vi "Dashboard Main.vi"() -> ()   [LabVIEW 2020]
uses:
  <vilib>/event_ctls.llb/eventvkey.ctl
  <vilib>/Rock Robotics/Network Tables/NT Read Numeric Array.vi
  <vilib>/Rock Robotics/WPI/Dashboard/WPI_DashboardLogging Global.vi
panel:
  in  "Camera Settings Right":T1={"Frame Rate"=30, "Compression"=30, "Size"=1, "DB Camera Config"=FALSE} {"Frame Rate" scale=1.0..30.0; "Compression" scale=100.0..-1.0; "Size" items=["640x480", "320x240", "160x120"]}
  in  "Camera Name Right":string(combo)="No Camera Selection"
  out "Camera Perf":string
  in  "Camera Settings":T1={"Frame Rate"=30, "Compression"=30, "Size"=1, "DB Camera Config"=FALSE} {"Frame Rate" scale=1.0..30.0; "Compression" scale=100.0..-1.0; "Size" items=["640x480", "320x240", "160x120"]}
  in  "TCP":refnum<k5>
  in  "Rec Mode":enum32{"Stop", "Record", "Playback"}(radio)
  out "Robot IP":string
  out "Image Message":string="Timeout in Camera Communications"
  in  "Dashboard Tab":T2(tab)
  in  "Select Auto":string(combo)="Select Autonomous ..."
  out "NT Connection":bool
  out "MotorChart R":cluster{"Numeric":dbl, "Numeric":dbl}(graph)
  out "MotorChart L":cluster{"Numeric":dbl, "Numeric":dbl}(graph)
  out "MotorSliders R":cluster{"MotorSlide1":dbl, "MotorSlide2":dbl} {"MotorSlide2" scale=-1.0..1.0 scale format="%#_2e"; "MotorSlide1" scale=-1.0..1.0 scale format="%#_2e"}
  out "MotorSliders L":cluster{"MotorSlide1":dbl, "MotorSlide2":dbl} {"MotorSlide2" scale=-1.0..1.0 scale format="%#_2e"; "MotorSlide1" scale=-1.0..1.0 scale format="%#_2e"}
  out "Gyro":dbl(knob) scale=0.0..360.0
  out "JS1 Z":dbl(slide) scale=-1.0..1.0 scale format="%#_2e"
  out "JS1 Graph":cluster{"X":dbl, "Y":dbl}[](graph)
  out "JS1 Buttons":T3
  out "JS2 Z":dbl(slide) scale=-1.0..1.0 scale format="%#_2e"
  out "JS2 Graph":cluster{"X":dbl, "Y":dbl}[](graph)
  out "JS2 Buttons":T3
  out "Mode":T4(ring)=enum."Auto Disabled"
  out "Right Camera Perf":cluster{"Bandwidth (Mbps)":dbl, "FPS":dbl}
  out "Camera Image Right":T5(plugin-control)
  in  "DB/String 9":string
  in  "DB/String 8":string
  in  "DB/String 7":string
  in  "DB/String 6":string
  in  "DB/String 5":string
  in  "DB/String 4":string
  in  "DB/String 3":string
  in  "DB/String 2":string
  in  "DB/String 1":string
  in  "DB/String 0":string
  in  "DB/Slider 0":dbl(slide) scale=0.0..5.0
  in  "DB/Slider 1":dbl(slide) scale=0.0..5.0
  in  "DB/Slider 2":dbl(slide) scale=0.0..5.0
  in  "DB/Slider 3":dbl(slide) scale=0.0..5.0
  out "DB/LED 3":bool
  out "DB/LED 2":bool
  out "DB/LED 1":bool
  out "DB/LED 0":bool
  in  "DB/Button 3":bool
  in  "DB/Button 2":bool
  in  "DB/Button 1":bool
  in  "DB/Button 0":bool caption="New Name"
  in  "Test Slider":dbl(slide) scale=0.0..100.0 scale format="%#_3g"
  in  "On/Off":bool caption="Solenoid"
  in  "Test Name":u16(ring) items=["Select the test to run..."]
  in  "Test Tree":string(tree)
  in  "Motor":cluster{"Value":dbl, "Enable":bool} {"Value" scale=-1.0..1.0 scale format="%#_3g"}
  out "Progress":T6 {"Test Progress" scale=0.0..100.0}
  in  "Rev/Fwd":cluster{"Forward":bool, "Reverse":bool}
  in  "Test Ring":u16(ring) items=["Monochrome", "Color"]
  in  "CheckList":i32(listbox)
  out "Tree":string(tree)
  out "XY Graph":cluster{"X":dbl, "Y":dbl}[](graph)
  out "Auto Step":T7 {"Arm"."Position" items=["PICKUP", "A", "B", "C"]; "Arm"."Direction" items=["NOTHING", "IN", "OUT"]}
  in  "Auto Steps":i32[](listbox)
  out "Auto Name":string
  out "Confirm Auto Selection":string
  out "Current Step":string
  in  "Auto Definitions":enum32{"Red 1", "Red 2"}(tab)
  in  "Red 1":T8(array[cluster]) {"Arm"."Position" items=["PICKUP", "A", "B", "C"]; "Arm"."Direction" items=["NOTHING", "IN", "OUT"]}
  in  "Red 2":T8(array[cluster]) {"Arm"."Position" items=["PICKUP", "A", "B", "C"]; "Arm"."Direction" items=["NOTHING", "IN", "OUT"]}
  in  "path to PNG file":path
  out "Formatted Strings":cluster{"Name":string, "Value":string}[](array[cluster])
  out "Camera Image":T5(plugin-control)
  out "Background":bool
  in  "Camera Name":string(combo)="No Camera Selection"
  # "HW"
  # "HW"
  # "Joysticks"
  # "Drive Motors"
  # "Front"
  # "Right"
  # "Left"
  # "Back"
  # "This tab is a great place for autonomous settings and robot-specific values.\nPlace controls and indicators inside this tab and match name to\nDashboard Variables on robot. You can also delete this comment."
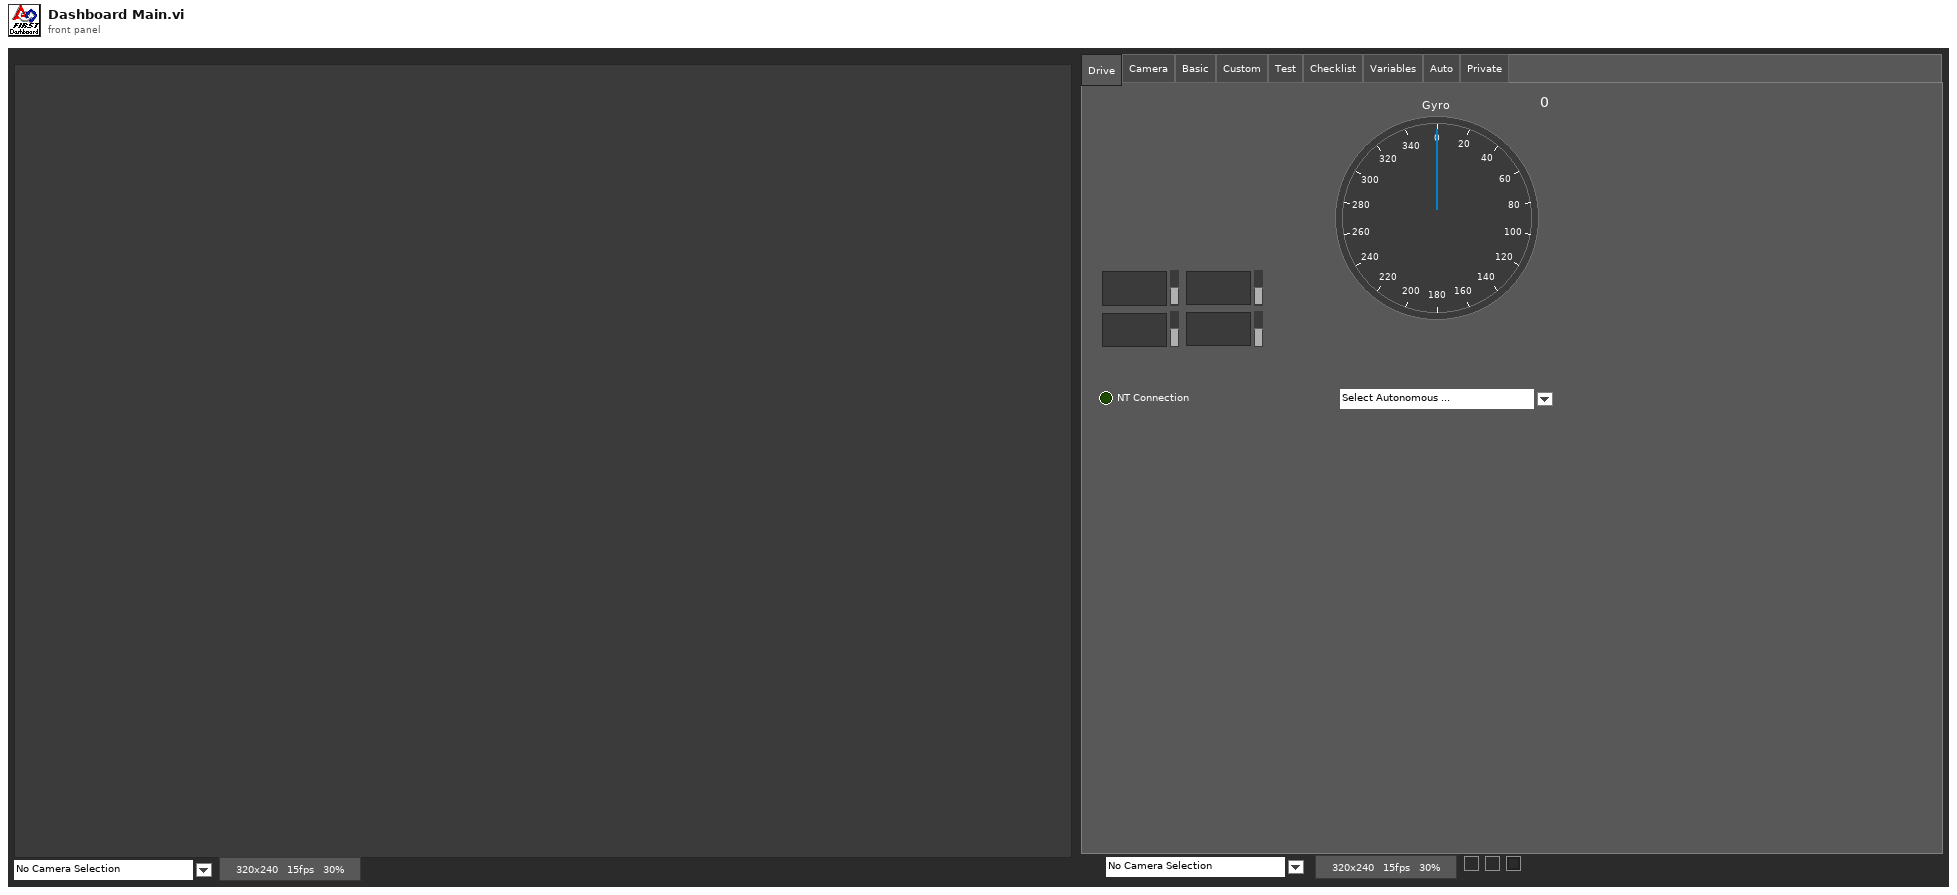
[diagram p1: front panel]
types:
  T1 = cluster{"Frame Rate":i32, "Compression":i32, "Size":u16, "DB Camera Config":bool}
  T2 = enum32{"Drive", "Camera", "Basic", "Custom", "Test", "Checklist", "Variables", "Auto", "Private"}
  T3 = cluster{bool, bool, bool, bool, bool, bool, bool, bool, bool, bool, bool, bool}
  T4 = enum8{"Tele-Op Disabled", "Tele-Op Enabled", "Auto Disabled", "Auto Enabled", "Test Disabled", "Test Enabled", "Disconnected", "No Code", "E-Stop"}
  T5 = typedef "IMAQ Image.ctl" = refnum<image>
  T6 = cluster{"Test Progress":u8, "Test Progress Text":string}
  T7 = cluster{"Step Name":string, "Position Change":cluster{"X":dbl, "Y":dbl, "Rotation":dbl, "Speed":dbl}, "Arm":cluster{"Direction":u16, "Position":u16}}
  T8 = cluster{"Step Name":string, "Position Change":cluster{"X":dbl, "Y":dbl, "Rotation":dbl, "Speed":dbl}, "Arm":cluster{"Direction":u16, "Position":u16}}[]
  T9 = enum32{"Drive", "Camera", "Basic", "Custom", "Test", "Checklist", "Variables"}
  T10 = cluster{"Save Path":path, "Interval (s)":dbl, "Keep":i32}
  T11 = enum32{"Drive", "Camera", "Basic", "Custom", "Test", "Commands", "Checklist", "Variables"}
  T12 = typedef "Image Type" = u32
  T13 = cluster{"Error Strings":string, "Disable Counts":cluster{u16, u16}, "Rail Faults":cluster{u16, u16, u16}, "Robot IP":string, "DB Mode":u8, "Event Info":cluster{"Name":string, "Type":u8, "Number":u16, "Replay":u8}}
  T14 = cluster{"Storage":cluster{"Disk Free":u64, "RAM Block":u32, "RAM free":u32}, "CPU Utilization":cluster{"CPU % ISR":sgl, "CPU % Time Crit":sgl, "CPU % Timed Str":sgl, "CPU % High":sgl, "CPU % Above":sgl, "CPU % Normal":sgl, "CPU % Low":sgl}, "CAN":cluster{"% Bus Utilization":sgl, "Bus Off Cnt":u32, "TX_FIFO Full Cnt":u32, "Receive Error Cnt":u8, "Transmit Error Cnt":u8}, "HID":cluster{"HID Outputs":u32, "Rumble Low":u16, "Rumble High":u16}[]}
  T15 = cluster{"Status bits":cluster{"Test Mode":bool, "Autonomous":bool, "Enabled":bool, "Code Start":bool, "Brownout":bool, "Reserved 2":bool, "Reserved 3":bool, "E-Stop":bool}, "Code Trace":cluster{"Disabled":bool, "TeleOp":bool, "Auto":bool, "Test":bool}, "Controller Type":enum16{"unknown", "cRIO", "roboRio"}, "Code?":enum16{"unknown", "noCode", "code"}, "Battery V":dbl}
  T16 = cluster{"Control Bits":cluster{"TestMode":bool, "Autonomous":bool, "Enabled":bool, "FMS Present":bool, bool, bool, bool, "E-Stop":bool}, "Team Station ":u8, "Countdown":sgl, "Joystick Values":cluster{"Axes":dbl[], "Buttons":bool[], "POVs":i16[]}[]}
  T17 = cluster{"Axes":dbl[], "Buttons":bool[], "POVs":i16[]}[]
  T18 = cluster{"Axes":dbl[], "Buttons":bool[], "POVs":i16[]}
  T19 = cluster{"Buttons[0]":bool, "Buttons[1]":bool, "Buttons[2]":bool, "Buttons[3]":bool, "Buttons[4]":bool, "Buttons[5]":bool, "Buttons[6]":bool, "Buttons[7]":bool, "Buttons[8]":bool, "Buttons[9]":bool, "Buttons[10]":bool, "Buttons[11]":bool}
  T20 = cluster{"Camera Image":refnum<vi>, "Dashboard Tab":refnum<vi>, "Background":refnum<vi>, "Rec Mode":refnum<vi>, "Test Slider":refnum<vi>, "On/Off ":refnum<vi>, "Test Ring":refnum<vi>, "Rev/Fwd":refnum<vi>, "Test Name":refnum<vi>, "Motor":refnum<vi>, "Progress":refnum<vi>, "CheckList":refnum<vi>, "Tree":refnum<vi>, "Test Tree":refnum<vi>, "Camera Settings":refnum<vi>, "Camera Name":refnum<vi>, "Camera Perf":refnum<vi>, "Camera Settings Right":refnum<vi>, "Camera Name Right":refnum<vi>, "Camera Image Right":refnum<vi>}
  T21 = cluster{"Global Rectangle":i32[], "Contours":cluster{"Contour Type":u32, "ROI Type":u32, "Points":i32[]}[]}
  T22 = cluster{"Camera Name":string, string, "Saved DB Images Info":cluster{"Save Path":path, "Interval (s)":dbl, "Keep":i32}}
  T23 = cluster{"Camera Name Right":string, string, "Saved DB Images Info":cluster{"Save Path":path, "Interval (s)":dbl, "Keep":i32}}
  T24 = cluster{"X":dbl, "Y":dbl, "Rotation":dbl, "Speed":dbl}
  T25 = cluster{"Operation":enum16{"Update", "Clear"}, "Color Box":u32}[]
  T26 = typedef "eventvkey.ctl" = enum16{"ASCII", "Enter", "Return", "Shift", "Ctrl", "Alt", "Cmd", "Opt", "Caps", "NumLock", "Clear", "Break", "Up", "Down", "Left", "Right", "Insert", "Delete", "Home", "End", "PageUp", "PageDown", "Escape", "Help", "Pause", "ScrollLock", "F1", "F2", "F3", "F4", "F5", "F6", "F7", "F8", "F9", "F10", "F11", "F12", "F13", "F14", "F15", "F16", "F17", "F18", "F19", "F20", "F21", "F22", "F23", "F24", "Play", "VolumeUp", "VolumeDown", "Mute", "Two Byte Char"}
  T27 = cluster{"Image Size":bool, "Image Type":bool, "Pixel Value":bool, "ROI Information":bool, "Zoom Factor":bool}
  T28 = cluster{"Operation":enum16{"Update", "Clear"}, "Color Box":u32}
  T29 = cluster{"Shift":bool, "Ctrl":bool, "Alt":bool, "Cmd":bool, "Opt":bool}
  T30 = typedef "imagedata.ctl" = cluster{"image type":i32, "image depth":i32, "image":u8[], "mask":u8[], "colors":u32[], "Rectangle":cluster{"left":i16, "top":i16, "right":i16, "bottom":i16}}
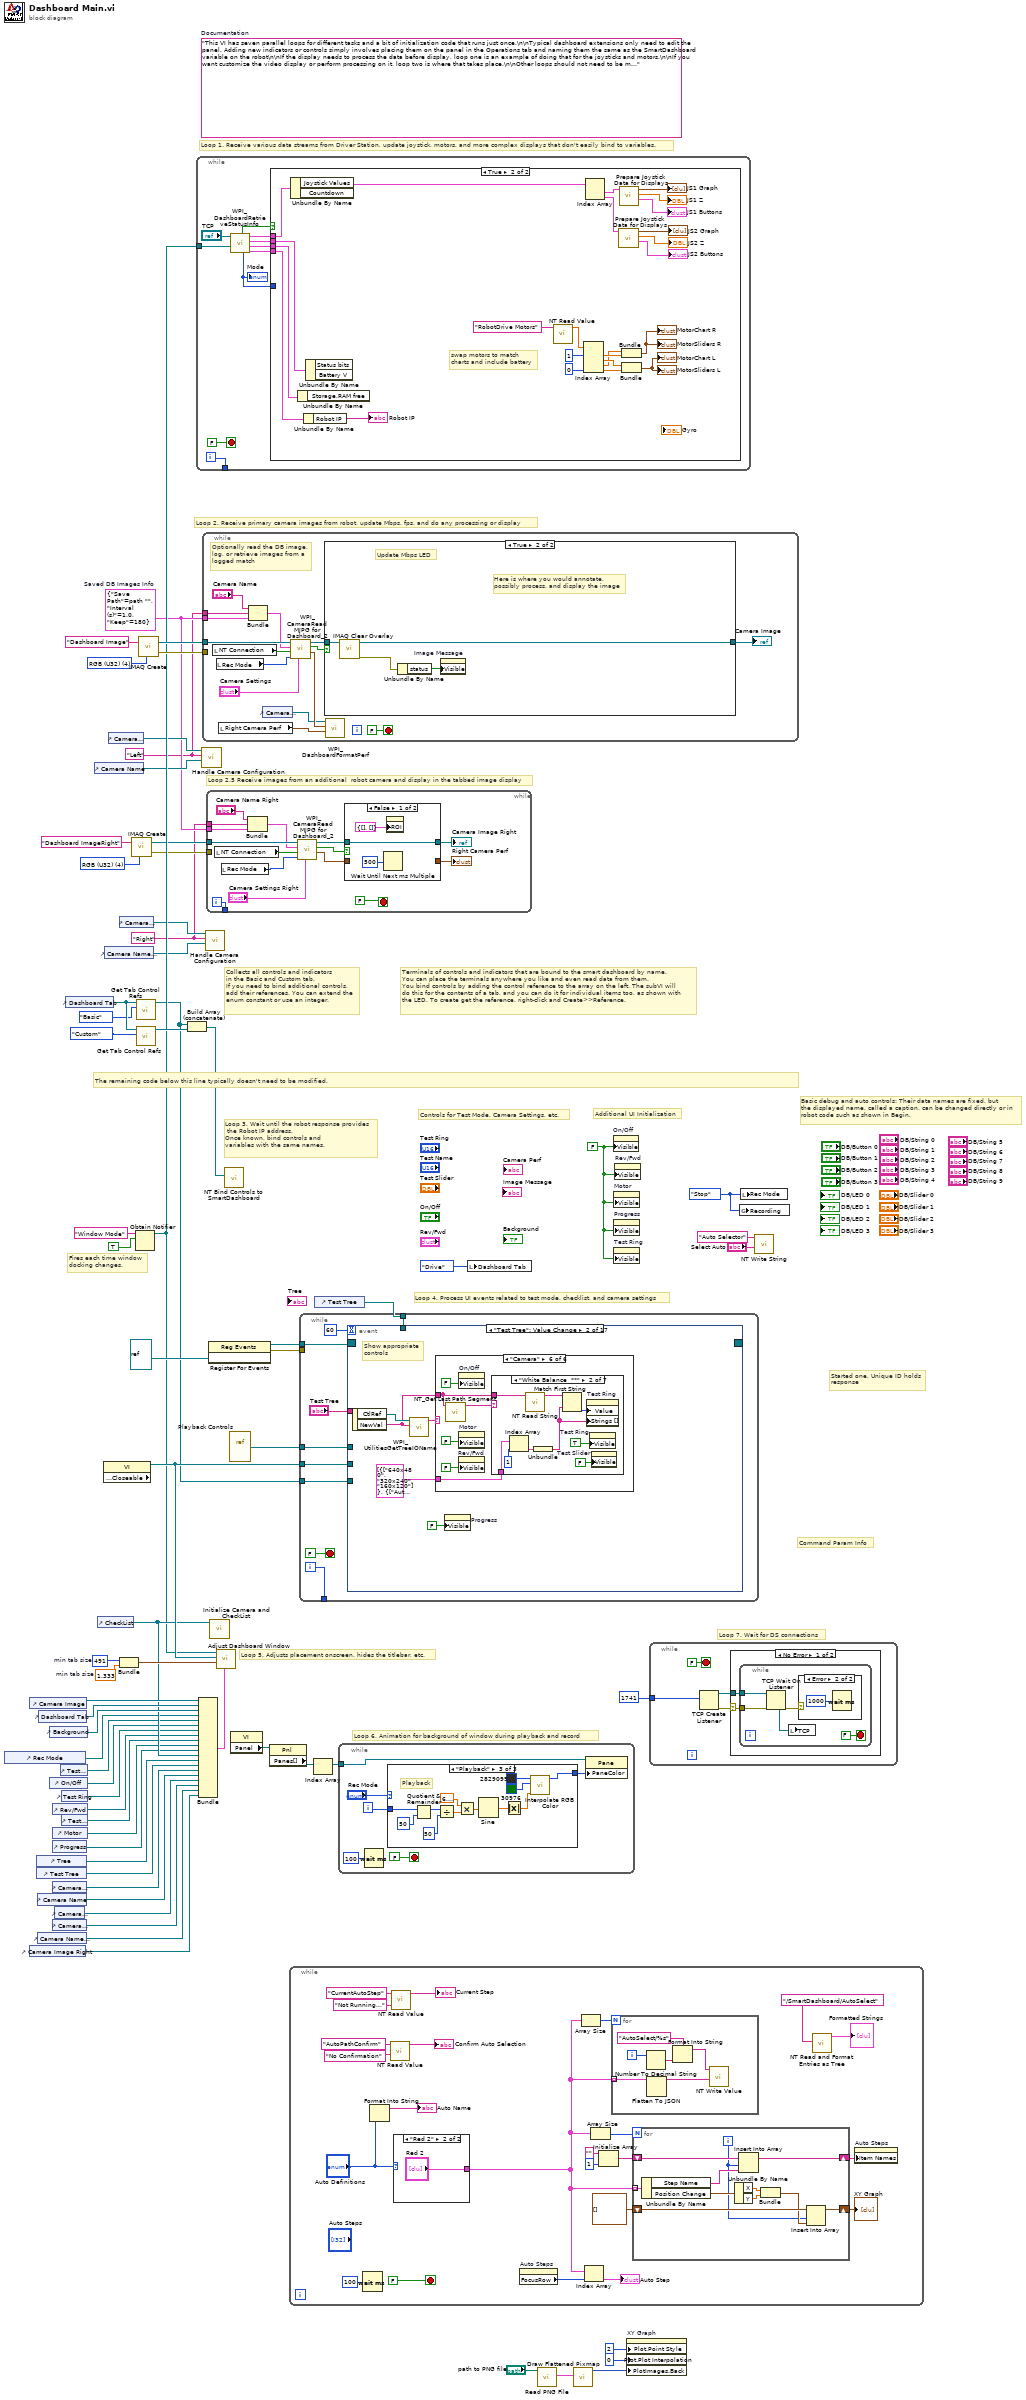
[diagram p0: block diagram]
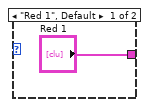
[diagram p2: hidden frame]
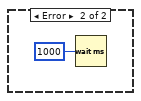
[diagram p5: hidden frame]
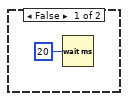
[diagram p6: hidden frame]
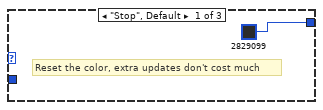
[diagram p7: hidden frame]
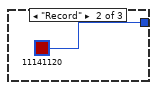
[diagram p8: hidden frame]
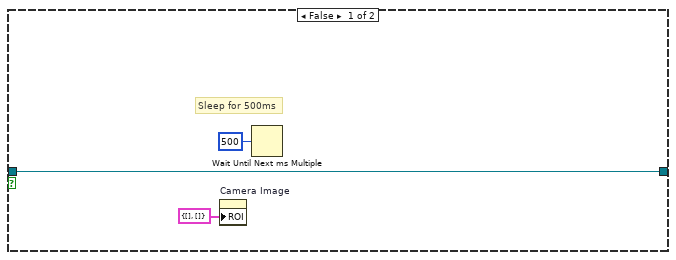
[diagram p9: hidden frame]
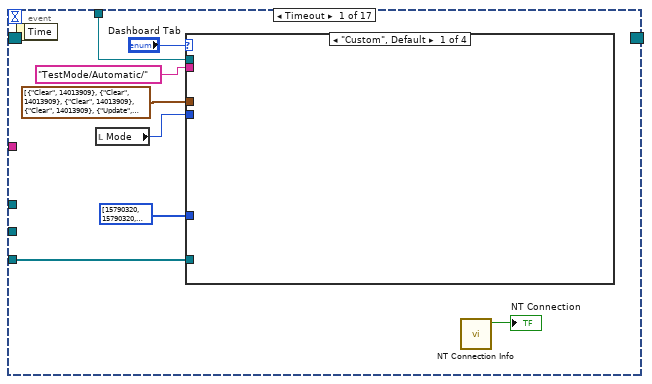
[diagram p10: hidden frame]
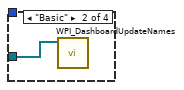
[diagram p11: hidden frame]
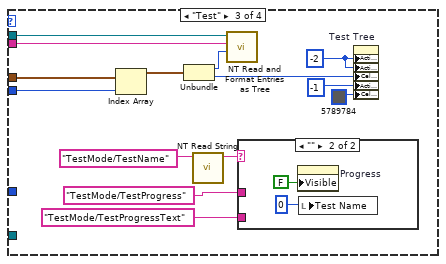
[diagram p12: hidden frame]
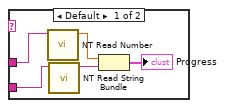
[diagram p13: hidden frame]
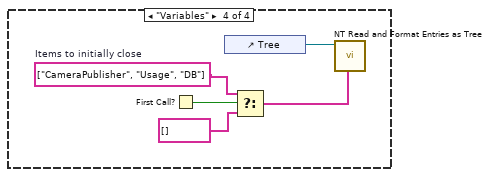
[diagram p14: hidden frame]
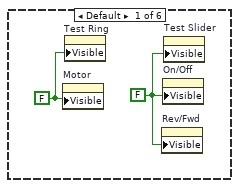
[diagram p15: hidden frame]
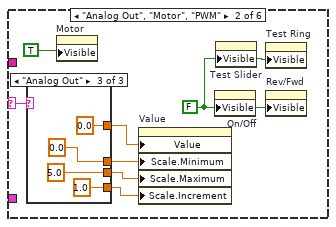
[diagram p16: hidden frame]
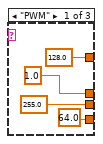
[diagram p17: hidden frame]
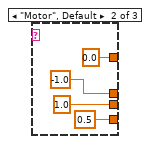
[diagram p18: hidden frame]
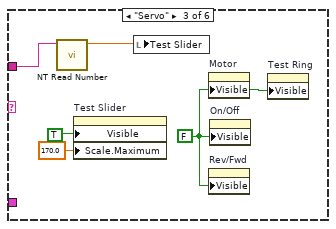
[diagram p19: hidden frame]
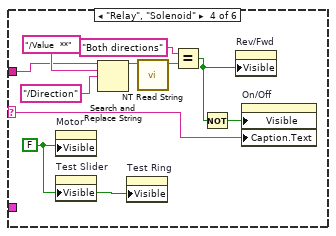
[diagram p20: hidden frame]
diagram:
  w8 = T10 {"Save Path"=path "", "Interval (s)"=1.0, "Keep"=180}  # Saved DB Images Info
  w7 = "Right"
  w6 = "Left"
  w18 = T12 4 items=["Grayscale (U8)", "Grayscale (I16)", "Grayscale (SGL)", "Complex (CSG)", "RGB (U32)", "HSL (U32)", "RGB (U64)"] ("Image Type")
  w47 = 491  # min tab size
  w46 = 1.333  # min tab size
  w54 = enum32{"Stop", "Record", "Playback"}."Stop" ("Rec Mode")
  w31 = FALSE ("Visible")
  (unwired) "This VI has seven parallel loops for different tasks and a bit of initialization code that runs just once.\n\nTypical dashboard extensions only need to edit the panel. Adding new indicators or controls simply involves placing them on the panel in the Operations tab and naming them the same as the SmartDashboard variable on the robot\n\nIf the display needs to process the data before display, loop one is an example of doing that for the joysticks and motors.\n\nIf you want customize the video display or perform processing on it, loop two is where that takes place.\n\nOther loops should not need to be modified. They are pretty standard, and document the task they perform."  # Documentation
  w68 = T12 4 items=["Grayscale (U8)", "Grayscale (I16)", "Grayscale (SGL)", "Complex (CSG)", "RGB (U32)", "HSL (U32)", "RGB (U64)"] ("Image Type")
  # "Loop 2.5 Receive images from an additional  robot camera and display in the tabbed image display"
  # "Command Param Info"
  # "Started one, Unique ID holds\nresponse"
  # "Loop 7. Wait for DS connections"
  # "Basic debug and auto controls: Their data names are fixed, but\nthe displayed name, called a caption, can be changed directly or in\nrobot code such as shown in Begin."
  # "Controls for Test Mode, Camera Settings, etc."
  # "Additional UI Initialization"
  # "Loop 6. Animation for background of window during playback and record"
  # "Fires each time window\ndocking changes."
  # "Collects all controls and indicators\nin the Basic and Custom tab.\nIf you need to bind additional controls,\nadd their references. You can extend the\nenum constant or use an integer."
  # "The remaining code below this line typically doesn't need to be modified."
  # "Loop 4. Process UI events related to test mode, checklist, and camera settings"
  # "Terminals of controls and indicators that are bound to the smart dashboard by name.\nYou can place the terminals anywhere you like and even read data from them.\nYou bind controls by adding the control reference to the array on the left. The subVI will\ndo this for the contents of a tab, and you can do it for individual items too, as shown with\nthe LED. To create get the reference, right-click and Create>>Reference."
  # "Loop 3. Wait until the robot response provides\n the Robot IP address.\nOnce known, bind controls and\nvariables with the same names."
  # "Loop 5. Adjusts placement onscreen, hides the titlebar, etc."
  # "Loop 1. Receive various data streams from Driver Station, update joystick, motors, and more complex displays that don't easily bind to variables."
  # "Loop 2. Receive primary camera images from robot, update Mbps, fps, and do any processing or display"
  n1 = control-ref of="Rec Mode"() -> (w37:refnum<vi>)
  n2 = control-ref of="Camera Image Right"() -> (w11:refnum<vi>)
  n3 = control-ref of="Camera Image"() -> (w49:refnum<vi>)
  n4 = control-ref of="Tree"() -> (w41:refnum<vi>)
  n5 = control-ref of="Test Tree"() -> (w40:refnum<vi>)
  n6 = control-ref of="Camera Name"() -> (w24:refnum<vi>)
  n7 = control-ref of="Camera Name Right"() -> (w12:refnum<vi>)
  n8 = control-ref of="Dashboard Tab"() -> (w48:refnum<vi>)
  n9 = control-ref of="Background"() -> (w44:refnum<vi>)
  n10 = control-ref of="On/Off"() -> (w35:refnum<vi>)
  n11 = control-ref of="Progress"() -> (w32:refnum<vi>)
  n12 = control-ref of="Camera Settings"() -> (w25:refnum<vi>)
  n13 = control-ref of="Camera Settings Right"() -> (w13:refnum<vi>)
  n14 = control-ref of="Rev/Fwd"() -> (w33:refnum<vi>)
  n15 = control-ref of="Motor"() -> (w38:refnum<vi>)
  n16 = control-ref of="Camera Perf"() -> (w23:refnum<vi>)
  n17 = control-ref of="Test Slider"() -> (w36:refnum<vi>)
  n18 = control-ref of="Test Ring"() -> (w34:refnum<vi>)
  n19 = control-ref of="Test Name"() -> (w39:refnum<vi>)
  n20 = control-ref of="Dashboard Tab"() -> (w52:refnum<vi>)
  n21 = control-ref of="Camera Name"() -> (w26:refnum<vi>)
  n22 = control-ref of="CheckList"() -> (w42:refnum<vi>)
  n23 = property class="VI" props=["Front Panel.Closeable"]() -> (reference out=w53:refnum<vi>)  [unwired: 2 in, 2 out]
  n24 = control-ref of="Camera Name Right"() -> (w14:refnum<vi>)
  n25 = control-ref of="Camera Settings"() -> (w27:refnum<vi>)
  n26 = control-ref of="Camera Settings Right"() -> (w15:refnum<vi>)
  n27 = Bundle("min tab size"=w47, "min tab size"=w46) -> (w45:cluster{"min tab size":i32, "min tab size":dbl})  [unwired: 1 in]
  n28 = call "IMAQ Create"("Image Name"="Dashboard ImageRight", "Image Type"=w18) -> ("New Image"=w17:T5, "error out"=w16:errorcluster)  [unwired: 2 in, 1 out]
  n29 = Obtain Notifier(name (unnamed)="Window Mode", notification data type=TRUE) -> (notifier out=w30:refnum<notifier>)  [unwired: 2 in, 2 out]
  n30 = call <vilib>:"Get Tab Control Refs.vi"("Page Index"=T11."Basic" ("Dashboard Tab"), "TabControl in"=w52) -> ("ControlsOnPage"=w22:refnum<vi>[])  [unwired: 9 in]
  n31 = call <vilib>:"Get Tab Control Refs.vi"("Page Index"=T11."Custom" ("Dashboard Tab"), "TabControl in"=w52) -> ("ControlsOnPage"=w51:refnum<vi>[])  [unwired: 9 in]
  n32 = call "IMAQ Create"("Image Name"="Dashboard Image", "Image Type"=w68) -> ("New Image"=w66:T5, "error out"=w65:errorcluster)  [unwired: 2 in, 1 out]
  n33 = Build Array (concatenate)(w22, w51) -> (w50:refnum<vi>[])
  n34 = while {
    tunnel: [w77] -> _
    tunnel: w30 -> [w69]
    i -> [w77]
    stop <- FALSE stop-if-true
    n35 = call <vilib>:"WPI_DashboardRetrieveStatusInfo.vi"("Window Mode Notifier"=w69, "TCP Cnx"="TCP") -> ("Power and Errors"=w72:T13, "Robot Metrics"=w75:T14, "Status Info"=w76:T15, "Control Info"=w73:T16, "Robot Mode"=w71:T4, "Process?"=w74:bool)  [unwired: 4 in]
    "Mode" <- w71
    n36 = case shown="True" w74 {
      tunnel: w76 -> [_ w103]
      tunnel: w75 -> [_ w102]
      tunnel: w73 -> [_ w101]
      tunnel: w72 -> [_ w100]
      tunnel: w71 -> [_ _]
      frame False {
        n37 = Wait (ms)(milliseconds to wait=u32 20) -> ()  [unwired: 1 out]
      }
      frame True {
        # "swap motors to match\ncharts and include battery"
        n38 = Unbundle By Name(w101) -> ("Joystick Values"=w91:T17)  [unwired: 1 out]
        n39 = Unbundle By Name(w102) -> ()  [unwired: 1 out]
        n40 = Unbundle By Name(w100) -> ("Robot IP"=→"Robot IP":string)
        n41 = Unbundle By Name(w103) -> ()  [unwired: 2 out]
        n42 = call-poly <vilib>:"NT Read Value.vi"("name"="RobotDrive Motors" ("Name")) -> ("value"=w81:dbl[])  [unwired: 8 in, 2 out]
        n43 = Index Array(array=w81, index #1=1, index #4=0) -> (element #1=w95:dbl, element #2=w96:dbl, element #3=w94:dbl, element #4=w99:dbl)  [unwired: 2 in]
        n44 = Index Array(array=w91) -> (element #1=w90:T18, element #2=w86:T18)  [unwired: 2 in]
        n45 = call "Prepare Joystick Data for Displays.vi"("Joystick Values"=w86) -> ("Buttons"=→"JS2 Buttons":T19, "Z Axis"=→"JS2 Z":dbl, "Cartesian Data"=→"JS2 Graph":cluster{"X axis":dbl, "X axis":dbl}[])  [unwired: 8 in]
        n46 = call "Prepare Joystick Data for Displays.vi"("Joystick Values"=w90) -> ("Buttons"=→"JS1 Buttons":T19, "Z Axis"=→"JS1 Z":dbl, "Cartesian Data"=→"JS1 Graph":cluster{"X axis":dbl, "X axis":dbl}[])  [unwired: 8 in]
        n47 = Bundle("Numeric"=w94, "Numeric"=w95) -> (→"MotorChart R" →"MotorSliders R":cluster{"Numeric":dbl, "Numeric":dbl})  [unwired: 1 in]
        n48 = Bundle("Numeric"=w96, "Numeric"=w99) -> (→"MotorChart L" →"MotorSliders L":cluster{"Numeric":dbl, "Numeric":dbl})  [unwired: 1 in]
      }
    }
  }
  n49 = Bundle("Camera Image"=w49, "Dashboard Tab"=w48, "Background"=w44, "Rec Mode"=w37, "Test Slider"=w36, "On/Off"=w35, "Test Ring"=w34, "Rev/Fwd"=w33, "Test Name"=w39, "Motor"=w38, "Progress"=w32, "CheckList"=w42, "Tree"=w41, "Test Tree"=w40, "Camera Settings"=w25, "Camera Name"=w24, "Camera Perf"=w23, "Camera Settings Right"=w13, "Camera Name Right"=w12, "Camera Image Right"=w11) -> (w43:T20)  [unwired: 1 in]
  n50 = call "Handle Camera Configuration.vi"("CameraNameRef"=w26, "Display Name"=w6, "ClusterRef"=w27) -> ()  [unwired: 9 in]
  n51 = while {
    tunnel: w66 -> [w117]
    tunnel: w65 -> [_]
    tunnel: w8 -> [w110]
    tunnel: w6 -> [w107]
    stop <- FALSE stop-if-true
    # "Optionally read the DB image,\nlog, or retrieve images from a\nlogged match"
    n52 = local read "NT Connection"() -> (w111:bool)
    n53 = local read "Rec Mode"() -> (w114:enum32{"Stop", "Record", "Playback"})
    n54 = local read "Right Camera Perf"() -> (w105:cluster{"Bandwidth (Mbps)":dbl, "FPS":dbl})
    n55 = Bundle("Camera Name"="Camera Name", w107, "Saved DB Images Info"=w110) -> (w109:T22)  [unwired: 1 in]
    n56 = control-ref of="Camera Perf"() -> (w104:refnum<vi>)
    n57 = call <vilib>:"WPI_CameraRead MJPG for Dashboard_2.vi"("Camera Settings"="Camera Settings", "Rec Mode"=w114, "NT Connection"=w111, "Capture Info"=w109, "Image in"=w117) -> ("perf info"=w106:cluster{"Bandwidth (Mbps)":dbl, "fps":dbl}, "Active"=w115:bool, "Image\\ out"=w116:T5)  [unwired: 4 in]
    n58 = case shown="True" w115 {
      tunnel: w116 -> [w120 w123]
      tunnel: [w120 w122] -> w112
      frame False {
        # "Sleep for 500ms"
        n59 = property on="Camera Image" class="ImageControl"("ROI"=T21 {"Global Rectangle"=[], "Contours"=[]}) -> ()  [unwired: 2 in, 2 out]
        n60 = Wait Until Next ms Multiple(millisecond multiple=u32 500) -> ()  [unwired: 1 out]
      }
      frame True {
        # "Here is where you would annotate,\npossibly process, and display the image"
        # "Update Mbps LED"
        n61 = call "IMAQ Clear Overlay"("Image"=w123) -> ("error out"=w124:errorcluster, "Image Out"=w122:T5)  [unwired: 2 in, 7 out]
        n62 = Unbundle By Name(w124) -> ("status"=w125:bool)
        n63 = property on="Image Message" class="Str"("Visible"=w125) -> ()  [unwired: 2 in, 2 out]
      }
    }
    "Camera Image" <- w112
    n64 = call <vilib>:"WPI_DashboardFormatPerf.vi"("Right Camera Perf"=w105, "Performance"=w106, "String in"=w104) -> ()  [unwired: 9 in]
  }
  n65 = call "Handle Camera Configuration.vi"("CameraNameRef"=w14, "Display Name"=w7, "ClusterRef"=w15) -> ()  [unwired: 9 in]
  n66 = while {
    tunnel: w17 -> [w140]
    tunnel: w16 -> [_]
    tunnel: [w135] -> _
    tunnel: w8 -> [w131]
    tunnel: w7 -> [w128]
    i -> [w135]
    stop <- FALSE stop-if-true
    n67 = local read "NT Connection"() -> (w132:bool)
    n68 = local read "Rec Mode"() -> (w139:enum32{"Stop", "Record", "Playback"})
    n69 = Bundle("Camera Name Right"="Camera Name Right", w128, "Saved DB Images Info"=w131) -> (w130:T23)  [unwired: 1 in]
    n70 = call <vilib>:"WPI_CameraRead MJPG for Dashboard_2.vi"("Camera Settings"="Camera Settings Right", "Rec Mode"=w139, "NT Connection"=w132, "Capture Info"=w130, "Image in"=w140) -> ("perf info"=w126:cluster{"Bandwidth (Mbps)":dbl, "fps":dbl}, "Active"=w134:bool, "Image\\ out"=w137:T5)  [unwired: 4 in]
    n71 = case shown="False" w134 {
      tunnel: w137 -> [w142 w145]
      tunnel: [w142 w145] -> w133
      tunnel: [_ w144] -> w127
      tunnel: w126 -> [_ w144]
      frame False {
        n72 = Wait Until Next ms Multiple(millisecond multiple=u32 500) -> ()  [unwired: 1 out]
        n73 = property on="Camera Image Right" class="ImageControl"("ROI"=T21 {"Global Rectangle"=[], "Contours"=[]}) -> ()  [unwired: 2 in, 2 out]
      }
      frame True {
      }
    }
    "Camera Image Right" <- w133
    "Right Camera Perf" <- w127
  }
  n74 = register-events(refnum<vi> refnum) -> (reference out=w57:refnum<event-registration>, error out=w56:errorcluster)  [unwired: 2 in]
  n75 = call "Initialize Camera and CheckList.vi"("ListBox in"=w42) -> ()  [unwired: 11 in]
  n76 = call "Adjust Dashboard Window.vi"("Sizing Refnums"=w43, "Size Constraints"=w45, "VI"=w53, "WIn Mode"=w30) -> ()  [unwired: 8 in]
  n77 = call <vilib>:"NT Bind Controls to SmartDashboard.vi"("Bound Control Refs"=w50) -> ()  [unwired: 11 in]
  n78 = vi-ref "Playback Controls.vi"() -> (w58:refnum<vi>)
  n79 = property class="VI"() -> ("Panel"=w60:refnum<vi>)  [unwired: 2 in, 2 out]
  n80 = property class="Pnl"(reference=w60) -> ("Panes[]"=w61:refnum<vi>[])  [unwired: 1 in, 2 out]
  n81 = while {
    stop <- FALSE stop-if-true
    n82 = Wait (ms)(milliseconds to wait=u32 100) -> ()  [unwired: 1 out]
    n83 = Format Into String("Auto Definitions") -> (resulting string=→"Auto Name":string)  [unwired: 3 in, 1 out]
    n84 = call-poly <vilib>:"NT Read Value.vi"("default value"="No Confirmation", "name"="AutoPathConfirm") -> ("value"=→"Confirm Auto Selection":string)  [unwired: 7 in, 2 out]
    n85 = call-poly <vilib>:"NT Read Value.vi"("default value"="Not Running...", "name"="CurrentAutoStep") -> ("value"=→"Current Step":string)  [unwired: 7 in, 2 out]
    n86 = case shown="\"Red 2\"" "Auto Definitions" {
      tunnel: ["Red 1" "Red 2"] -> w154
      frame "Red 1", Default {
      }
      frame "Red 2" {
      }
    }
    n87 = property on="Auto Steps" class="LstBox (strict)"() -> ("FocusRow"=w159:i32)  [unwired: 2 in, 2 out]
    n88 = Array Size(array=w154) -> (size(s)=w168:i32)
    n89 = Index Array(array=w154, index=w159) -> (element=→"Auto Step":T7)
    n90 = Array Size(array=w154) -> (size(s)=w163:i32)
    n91 = Initialize Array("" ("element"), 1 ("dimension size")) -> (w162:string[])
    n92 = for {
      N: w168 -> [_]
      tunnel: w154 -> [w187] mode=indexing
      i -> [w183]
      n93 = Number To Decimal String(number=w183) -> (decimal integer string=w184:string)  [unwired: 1 in]
      n94 = Flatten To JSON(anything=w187) -> (JSON string=w186:string)  [unwired: 2 in, 1 out]
      n95 = Format Into String(format string="AutoSelect/%s", w184) -> (resulting string=w182:string)  [unwired: 2 in, 1 out]
      n96 = call-poly <vilib>:"NT Write Value.vi"("value"=w186, "name"=w182) -> ()  [unwired: 9 in, 1 out]
    }
    n97 = for {
      N: w163 -> [_]
      tunnel: w154 -> [w181] mode=indexing
      shift-right: [w179] -> w165
      shift-left: w162 -> [w180]
      shift-right: [w173] -> w156
      shift-left: cluster{"X":dbl, "Y":dbl}[] [] -> [w174]
      i -> [w171]
      n98 = Unbundle By Name(w181) -> ("Step Name"=w178:string, "Position Change"=w177:T24)
      n99 = Unbundle By Name(w177) -> ("X"=w175:dbl, "Y"=w176:dbl)
      n100 = Insert Into Array(array=w180, index=w171, new element=w178) -> (w179:string[])
      n101 = Bundle("X"=w175, "Y"=w176) -> (w172:cluster{"X":dbl, "Y":dbl})  [unwired: 1 in]
      n102 = Insert Into Array(array=w174, index=w171, new element=w172) -> (w173:cluster{"X":dbl, "Y":dbl}[])
    }
    "XY Graph" <- w156
    n103 = call <vilib>:"NT Read and Format Entries as Tree.vi"("Name Pattern"="/SmartDashboard/AutoSelect") -> ("Formatted Strings"=→"Formatted Strings":cluster{"Name":string, "Value":string}[])  [unwired: 9 in, 1 out]
    n104 = property on="Auto Steps" class="LstBox (strict)"("Item Names"=w165) -> ()  [unwired: 2 in, 2 out]
  }
  n105 = Index Array(array=w61) -> (element=w59:refnum<vi>)  [unwired: 1 in]
  n106 = control-ref of="Test Tree"() -> (w62:refnum<vi>)
  n107 = while {
    tunnel: [w193] -> _
    tunnel: w62 -> [w192]
    tunnel: w58 -> [w191]
    tunnel: w57 -> [w190]
    tunnel: w56 -> [_]
    tunnel: w53 -> [w189]
    tunnel: w22 -> [w188]
    i -> [w193]
    stop <- FALSE stop-if-true
    n108 = event shown="[1] \"Test Tree\": Value Change" {
      selector: w190 -> [_ _ _ _ _ _ _ _ _ _ _ _ _ _ _ _ _]
      dyn-events: [_ _ _ _ _ _ _ _ _ _ _ _ _ w398 _ _ _] -> _
      timeout: u32 60 ("milliseconds to wait") -> [_ _ _ _ _ _ _ _ _ _ _ _ _ _ _ _ _]
      tunnel: w192 -> [w203 _ _ _ _ _ _ _ _ _ _ _ _ _ _ _ _]
      tunnel: "Test Tree" -> [_ _ _ _ _ _ _ _ w371 w378 w379 w382 w389 _ _ _ _]
      tunnel: w191 -> [_ _ _ _ _ _ _ _ _ _ _ _ _ w400 _ w415 _]
      tunnel: w189 -> [_ _ _ _ _ _ _ _ _ _ _ _ _ w396 _ _ _]
      tunnel: w188 -> [w198 _ _ _ _ _ _ _ _ _ _ _ _ _ _ _ _]
      event Timeout {
        n109 = event-data() -> ()  [unwired: 1 in, 1 out]
        n110 = local read "Mode"() -> (w201:T4)
        n111 = case shown="\"Custom\", Default" "Dashboard Tab" {
          tunnel: w203 -> [_ _ w219 _]
          tunnel: "TestMode/Automatic/" ("Name Pattern") -> [_ _ w218 _]
          tunnel: T25 [{"Operation"=enum."Clear", "Color Box"=14013909}, {"Operation"=enum."Clear", "Color Box"=14013909}, {"Operation"=enum."Clear", "Color Box"=14013909}, {"Operation"=enum."Clear", "Color Box"=14013909}, {"Operation"=enum."Update", "Color Box"=14013909}, {"Operation"=enum."Update", "Color Box"=16777215}, {"Operation"=enum."Clear", "Color Box"=14013909}, {"Operation"=enum."Clear", "Color Box"=14013909}, {"Operation"=enum."Clear", "Color Box"=14013909}] -> [_ _ w211 _]
          tunnel: w201 -> [_ _ w210 _]
          tunnel: u32[] [15790320, 15790320, 15790320, 15790320, 16777215, 16777215, 15790320, 15790320, 15790320] -> [_ _ _ _]
          tunnel: w198 -> [_ w205 _ _]
          frame "Custom", Default {
          }
          frame "Basic" {
            n112 = call <vilib>:"WPI_DashboardUpdateNames.vi"("Controls on Tab"=w205) -> ()  [unwired: 11 in]
          }
          frame "Test" {
            w217 = -2 ("Active Item:Row Number")
            n113 = Index Array(array=w211, index=w210) -> (element=w212:T28)
            n114 = Unbundle(w212) -> ("Operation"=w213:enum16{"Update", "Clear"}, "Color Box"=w214:u32)
            n115 = call <vilib>:"NT Read String.vi"("name"="TestMode/TestName" ("Name")) -> ("value"=w208:string)  [unwired: 8 in, 2 out]
            n116 = call <vilib>:"NT Read and Format Entries as Tree.vi"("Operation"=w213, "Name Pattern"=w218, "Tree Refnum"=w219) -> ()  [unwired: 7 in, 2 out]
            n117 = case shown="\"\"" w208 {
              tunnel: "TestMode/TestProgress" ("Name") -> [w221 _]
              tunnel: "TestMode/TestProgressText" ("Name") -> [w220 _]
              frame Default {
                n118 = call <vilib>:"NT Read Number.vi"("name"=w221) -> ("value"=w222:dbl)  [unwired: 8 in, 2 out]
                n119 = call <vilib>:"NT Read String.vi"("name"=w220) -> ("value"=w223:string)  [unwired: 8 in, 2 out]
                n120 = Bundle("value"=w222, "value"=w223) -> (→"Progress":cluster{"value":dbl, "value":string})  [unwired: 1 in]
              }
              frame "" {
                n121 = property on="Progress" class="Clust (strict)"("Visible"=FALSE) -> ()  [unwired: 2 in, 2 out]
                n122 = local write "Test Name"(u16 0) -> ()
              }
            }
            n123 = property on="Test Tree" class="Tree (strict)"("Active Item Row Number"=w217, "ActiveColNum"=w217, "CellBG"=w214, "Active Item Row Number"=-1 ("Active Item:Row Number"), "CellBG"=u32 5789784 ("Color Box")) -> ()  [unwired: 2 in, 2 out]
          }
          frame "Variables" {
            w229 = string[] ["CameraPublisher", "Usage", "DB"]  # Items to initially close
            n124 = First Call?() -> (First Call?: T/F=w230:bool)
            n125 = control-ref of="Tree"() -> (w231:refnum<vi>)
            n126 = Select(t=w229, s=w230, f=string[] []) -> (s? t:f=w227:string[])
            n127 = call <vilib>:"NT Read and Format Entries as Tree.vi"("Tags to  Close"=w227, "Tree Refnum"=w231) -> ()  [unwired: 8 in, 2 out]
          }
        }
        n128 = call <vilib>:"NT Connection Info.vi"() -> ("Connected"=→"NT Connection":bool)  [unwired: 11 in]
      }
      event "Test Tree": Value Change {
        # "Show appropriate\ncontrols"
        n129 = event-data() -> ("CtlRef"=w235:refnum<vi>, "NewVal"=w233:string)  [unwired: 1 in]
        n130 = call <vilib>:"WPI_UtilitiesGetTreeIOName.vi"("NewVal"=w233, "TreeControl in"=w235) -> ("I/O Name"=w236:string)  [unwired: 9 in]
        n131 = case shown="\"Camera\"" w236 {
          selector: w236 -> [_ w243 _ w265 w274 _]
          tunnel: w233 -> [_ _ w262 w264 _ w281]
          tunnel: cluster{string[]}[] [{["640x480", "320x240", "160x120"]}, {["Auto", "Fixed indoor", "Fixed outdoor 1", "Fixed outdoor 2", "Fixed fluorescent 1", "Fixed fluorescent 2", "Hold current"]}, {["Auto", "Flicker-free 50 Hz", "Flicker-free 60 Hz", "Hold current"]}, {["None", "Prioritize frame rate", "Prioritize image quality"]}, {["Monochrome", "Color"]}] -> [_ _ _ _ _ w280]
          frame Default {
            w238 = FALSE ("Visible")
            w237 = FALSE ("Visible")
            n132 = property on="Motor" class="Clust (strict)"("Visible"=w237) -> ()  [unwired: 2 in, 2 out]
            n133 = property on="Test Ring" class="Ring (strict)"("Visible"=w237) -> ()  [unwired: 2 in, 2 out]
            n134 = property on="Rev/Fwd" class="Clust (strict)"("Visible"=w238) -> ()  [unwired: 2 in, 2 out]
            n135 = property on="On/Off" class="Bool (strict)"("Visible"=w238) -> ()  [unwired: 2 in, 2 out]
            n136 = property on="Test Slider" class="Slide (strict)"("Visible"=w238) -> ()  [unwired: 2 in, 2 out]
          }
          frame "Analog Out", "Motor", "PWM" {
            w244 = FALSE ("Visible")
            n137 = case shown="\"Analog Out\"" w243 {
              tunnel: [1.0 ("Value") -1.0 ("Value") 0.0 ("Value")] -> w242
              tunnel: [255.0 ("Value") 1.0 ("Value") 5.0 ("Value")] -> w241
              tunnel: [128.0 ("Value") 0.0 ("Value") 0.0 ("Value")] -> w240
              tunnel: [64.0 ("Value") 0.5 ("Value") 1.0 ("Value")] -> w239
              frame "PWM" {
              }
              frame "Motor", Default {
              }
              frame "Analog Out" {
              }
            }
            n138 = property on="Motor" class="Clust (strict)"("Visible"=TRUE) -> ()  [unwired: 2 in, 2 out]
            n139 = property on="Value" class="Slide (strict)"("Value"=w240, "Scale.Minimum"=w242, "Scale.Maximum"=w241, "Scale.Increment"=w239) -> ()  [unwired: 2 in, 2 out]
            n140 = property on="On/Off" class="Bool (strict)"("Visible"=w244) -> ()  [unwired: 2 in, 2 out]
            n141 = property on="Test Slider" class="Slide (strict)"("Visible"=w244) -> ()  [unwired: 2 in, 2 out]
            n142 = property on="Test Ring" class="Ring (strict)"("Visible"=w244) -> ()  [unwired: 2 in, 2 out]
            n143 = property on="Rev/Fwd" class="Clust (strict)"("Visible"=w244) -> ()  [unwired: 2 in, 2 out]
          }
          frame "Servo" {
            w260 = FALSE ("Visible")
            n144 = call <vilib>:"NT Read Number.vi"("name"=w262) -> ("value"=w261:dbl)  [unwired: 8 in, 2 out]
            n145 = property on="Test Slider" class="Slide (strict)"("Visible"=TRUE, "Scale.Maximum"=170.0 ("Scale.Range:Maximum")) -> ()  [unwired: 2 in, 2 out]
            n146 = local write "Test Slider"(w261) -> ()
            n147 = property on="Motor" class="Clust (strict)"("Visible"=w260) -> ()  [unwired: 2 in, 2 out]
            n148 = property on="Rev/Fwd" class="Clust (strict)"("Visible"=w260) -> ()  [unwired: 2 in, 2 out]
            n149 = property on="On/Off" class="Bool (strict)"("Visible"=w260) -> ()  [unwired: 2 in, 2 out]
            n150 = property on="Test Ring" class="Ring (strict)"("Visible"=w260) -> ()  [unwired: 2 in, 2 out]
          }
          frame "Relay", "Solenoid" {
            w263 = FALSE ("Visible")
            n151 = property on="Motor" class="Clust (strict)"("Visible"=w263) -> ()  [unwired: 2 in, 2 out]
            n152 = property on="Test Slider" class="Slide (strict)"("Visible"=w263) -> ()  [unwired: 2 in, 2 out]
            n153 = Search and Replace String(input string=w264, search string="/Value  **", replace string="/Direction") -> (result string=w270:string)  [unwired: 5 in, 3 out]
            n154 = property on="Test Ring" class="Ring (strict)"("Visible"=w263) -> ()  [unwired: 2 in, 2 out]
            n155 = call <vilib>:"NT Read String.vi"("name"=w270) -> ("value"=w268:string)  [unwired: 8 in, 2 out]
            n156 = Equal?(x="Both directions", y=w268) -> (x = y?=w266:bool)
            n157 = Not(x=w266) -> (.not. x?=w267:bool)
            n158 = property on="Rev/Fwd" class="Clust (strict)"("Visible"=w266) -> ()  [unwired: 2 in, 2 out]
            n159 = property on="On/Off" class="Bool (strict)"("Visible"=w267, "Caption.Text"=w265) -> ()  [unwired: 2 in, 2 out]
          }
          frame "Compressor", "Digital Out" {
            w273 = FALSE ("Visible")
            # "Get direction and finish"
            n160 = property on="Motor" class="Clust (strict)"("Visible"=w273) -> ()  [unwired: 2 in, 2 out]
            n161 = property on="Test Slider" class="Slide (strict)"("Visible"=w273) -> ()  [unwired: 2 in, 2 out]
            n162 = property on="Test Ring" class="Ring (strict)"("Visible"=w273) -> ()  [unwired: 2 in, 2 out]
            n163 = property on="On/Off" class="Bool (strict)"("Visible"=TRUE, "Caption.Text"=w274) -> ()  [unwired: 2 in, 2 out]
            n164 = property on="Rev/Fwd" class="Clust (strict)"("Visible"=FALSE) -> ()  [unwired: 2 in, 2 out]
          }
          frame "Camera" {
            n165 = call <vilib>:"NT_Get Last Path Segment.vi"("String in"=w281) -> ("String out"=w282:string)  [unwired: 10 in]
            n166 = property on="On/Off" class="Bool (strict)"("Visible"=FALSE) -> ()  [unwired: 2 in, 2 out]
            n167 = property on="Motor" class="Clust (strict)"("Visible"=FALSE) -> ()  [unwired: 2 in, 2 out]
            n168 = property on="Rev/Fwd" class="Clust (strict)"("Visible"=FALSE) -> ()  [unwired: 2 in, 2 out]
            n169 = case shown="\"White Balance  **\"" w282 {
              tunnel: w281 -> [w288 w297 w306 w315 w324 _ w330]
              tunnel: w280 -> [w286 w294 w303 w312 w321 _ _]
              frame "Size  **" {
                n170 = Index Array(array=w286) -> (element=w285:cluster{string[]})  [unwired: 1 in]
                n171 = call <vilib>:"NT Read String.vi"("name"=w288) -> ("value"=w287:string)  [unwired: 8 in, 2 out]
                n172 = Unbundle(w285) -> (w283:string[])
                n173 = Match First String(2:w283, 3:w287) -> (0:w284:i32)  [unwired: 1 out]
                n174 = property on="Test Ring" class="Ring (strict)"("Value"=w284, "Strings []"=w283) -> ()  [unwired: 2 in, 2 out]
                n175 = property on="Test Ring" class="Ring (strict)"("Visible"=TRUE) -> ()  [unwired: 2 in, 2 out]
                n176 = property on="Test Slider" class="Slide (strict)"("Visible"=FALSE) -> ()  [unwired: 2 in, 2 out]
              }
              frame "White Balance  **" {
                n177 = Index Array(array=w294, index=1) -> (element=w295:cluster{string[]})
                n178 = call <vilib>:"NT Read String.vi"("name"=w297) -> ("value"=w296:string)  [unwired: 8 in, 2 out]
                n179 = Unbundle(w295) -> (w292:string[])
                n180 = Match First String(2:w292, 3:w296) -> (0:w291:i32)  [unwired: 1 out]
                n181 = property on="Test Ring" class="Ring (strict)"("Value"=w291, "Strings []"=w292) -> ()  [unwired: 2 in, 2 out]
                n182 = property on="Test Ring" class="Ring (strict)"("Visible"=TRUE) -> ()  [unwired: 2 in, 2 out]
                n183 = property on="Test Slider" class="Slide (strict)"("Visible"=FALSE) -> ()  [unwired: 2 in, 2 out]
              }
              frame "Exposure  **" {
                n184 = Index Array(array=w303, index=2) -> (element=w304:cluster{string[]})
                n185 = call <vilib>:"NT Read String.vi"("name"=w306) -> ("value"=w305:string)  [unwired: 8 in, 2 out]
                n186 = Unbundle(w304) -> (w300:string[])
                n187 = Match First String(2:w300, 3:w305) -> (0:w301:i32)  [unwired: 1 out]
                n188 = property on="Test Ring" class="Ring (strict)"("Value"=w301, "Strings []"=w300) -> ()  [unwired: 2 in, 2 out]
                n189 = property on="Test Ring" class="Ring (strict)"("Visible"=TRUE) -> ()  [unwired: 2 in, 2 out]
                n190 = property on="Test Slider" class="Slide (strict)"("Visible"=FALSE) -> ()  [unwired: 2 in, 2 out]
              }
              frame "Exposure Priority  **" {
                n191 = Index Array(array=w312, index=3) -> (element=w313:cluster{string[]})
                n192 = call <vilib>:"NT Read String.vi"("name"=w315) -> ("value"=w314:string)  [unwired: 8 in, 2 out]
                n193 = Unbundle(w313) -> (w309:string[])
                n194 = Match First String(2:w309, 3:w314) -> (0:w310:i32)  [unwired: 1 out]
                n195 = property on="Test Ring" class="Ring (strict)"("Value"=w310, "Strings []"=w309) -> ()  [unwired: 2 in, 2 out]
                n196 = property on="Test Ring" class="Ring (strict)"("Visible"=TRUE) -> ()  [unwired: 2 in, 2 out]
                n197 = property on="Test Slider" class="Slide (strict)"("Visible"=FALSE) -> ()  [unwired: 2 in, 2 out]
              }
              frame "Color Enable  **" {
                n198 = Index Array(array=w321, index=4) -> (element=w322:cluster{string[]})
                n199 = call <vilib>:"NT Read String.vi"("name"=w324) -> ("value"=w323:string)  [unwired: 8 in, 2 out]
                n200 = Unbundle(w322) -> (w318:string[])
                n201 = Match First String(2:w318, 3:w323) -> (0:w319:i32)  [unwired: 1 out]
                n202 = property on="Test Ring" class="Ring (strict)"("Value"=w319, "Strings []"=w318) -> ()  [unwired: 2 in, 2 out]
                n203 = property on="Test Ring" class="Ring (strict)"("Visible"=TRUE) -> ()  [unwired: 2 in, 2 out]
                n204 = property on="Test Slider" class="Slide (strict)"("Visible"=FALSE) -> ()  [unwired: 2 in, 2 out]
              }
              frame Default {
                n205 = property on="Test Ring" class="Ring (strict)"("Visible"=FALSE) -> ()  [unwired: 2 in, 2 out]
                n206 = property on="Test Slider" class="Slide (strict)"("Visible"=FALSE) -> ()  [unwired: 2 in, 2 out]
              }
              frame "Brightness  **", "Color Level  **", "Compression  **", "FPS  **", "Sharpness  **" {
                n207 = call <vilib>:"NT Read Number.vi"("name"=w330) -> ("value"=w329:dbl)  [unwired: 8 in, 2 out]
                n208 = local write "Test Slider"(w329) -> ()
                n209 = property on="Test Slider" class="Slide (strict)"("Visible"=TRUE, "Scale.Maximum"=100.0 ("Scale.Range:Maximum")) -> ()  [unwired: 2 in, 2 out]
                n210 = property on="Test Ring" class="Ring (strict)"("Visible"=FALSE) -> ()  [unwired: 2 in, 2 out]
              }
            }
          }
        }
        n211 = property on="Progress" class="Clust (strict)"("Visible"=FALSE) -> ()  [unwired: 2 in, 2 out]
      }
      event "Test Name": Mouse Enter {
        # "Populate the ring with the list of tests"
        n212 = event-data() -> ()  [unwired: 1 in, 1 out]
        n213 = call <vilib>:"NT Read String Array.vi"("name"="TestMode/TestList" ("Name")) -> ("value"=w337:string[])  [unwired: 8 in, 2 out]
        n214 = Build Array (concatenate)("Select the test to run...", w337) -> (w336:string[])
        n215 = property on="Test Name" class="Ring (strict)"("Strings []"=w336) -> ()  [unwired: 2 in, 2 out]
      }
      event "Test Name": Value Change {
        w338 = FALSE ("Visible")
        # "Tell the robot the test name to run"
        n216 = event-data() -> ("NewVal"=w342:u16)  [unwired: 1 in]
        n217 = property on="Test Name" class="Ring (strict)"() -> ("Strings []"=w343:string[])  [unwired: 2 in, 2 out]
        n218 = local write "Progress"(T6 {"Test Progress"=0, "Test Progress Text"=""} ("Progress")) -> ()
        n219 = Index Array(array=w343, index=w342) -> (element=w341:string)
        n220 = call <vilib>:"NT Write String.vi"("value"=w341, "name"="TestMode/TestName" ("Name")) -> ()  [unwired: 9 in, 1 out]
        n221 = property on="Progress" class="Clust (strict)"("Visible"=TRUE) -> ()  [unwired: 2 in, 2 out]
        n222 = property on="Motor" class="Clust (strict)"("Visible"=w338) -> ()  [unwired: 2 in, 2 out]
        n223 = property on="Test Slider" class="Slide (strict)"("Visible"=w338) -> ()  [unwired: 2 in, 2 out]
        n224 = property on="On/Off" class="Bool (strict)"("Visible"=w338) -> ()  [unwired: 2 in, 2 out]
        n225 = property on="Rev/Fwd" class="Clust (strict)"("Visible"=w338) -> ()  [unwired: 2 in, 2 out]
        n226 = property on="Test Ring" class="Ring (strict)"("Visible"=w338) -> ()  [unwired: 2 in, 2 out]
      }
      event "Select Auto": Mouse Enter {
        # "Populate the combo box with the list of autonomous options"
        n227 = event-data() -> ()  [unwired: 1 in, 1 out]
        n228 = call <vilib>:"NT Read String Array.vi"("name"="Auto List" ("Name")) -> ("value"=w345:string[])  [unwired: 8 in, 2 out]
        n229 = property on="Select Auto" class="CmbBox"("Strings[]"=w345) -> ()  [unwired: 2 in, 2 out]
      }
      event "Select Auto": Value Change {
        # "User modified the Auto Selection. Write to NT variable so robot knows."
        n230 = event-data() -> ("NewVal"=w347:string)  [unwired: 1 in]
        n231 = call <vilib>:"NT Write String.vi"("value"=w347, "name"="Auto Selector" ("Name")) -> ()  [unwired: 9 in, 1 out]
      }
      event "CheckList": Double Click {
        # "Shift clears all"
        # "Update symbols on the listbox"
        n232 = event-data() -> ("PlatMods.Shift"=w349:bool, "Row"=w351:i32)  [unwired: 1 in]
        n233 = case shown="True" w349 {
          tunnel: w351 -> [w355 _]
          tunnel: 1 -> [w354 _]
          frame False {
            n234 = property on="CheckList" class="LstBox (strict)"() -> ("Item Symbols"=w353:i32[])  [unwired: 2 in, 2 out]
            n235 = Replace Array Subset(array=w353, new element=w354, index=w355) -> (w352:i32[])
            n236 = property on="CheckList" class="LstBox (strict)"("Item Symbols"=w352) -> ()  [unwired: 2 in, 2 out]
          }
          frame True {
            w356 = 0 ("Top Row")
            n237 = property on="CheckList" class="LstBox (strict)"() -> ("Number of Rows"=w358:u32)  [unwired: 2 in, 2 out]
            n238 = Initialize Array(0, w358) -> (w357:i32[])
            n239 = property on="CheckList" class="LstBox (strict)"("Top Row"=w356, "Value"=w356, "Item Symbols"=w357) -> ()  [unwired: 2 in, 2 out]
          }
        }
      }
      event "CheckList": Key Down {
        # "Update symbols on the listbox\nLeft and right keys check and uncheck"
        n240 = event-data() -> ("VKey"=w361:T26)  [unwired: 1 in]
        n241 = case shown="\"Left\", \"Right\"" w361 {
          selector: w361 -> [w366 _]
          tunnel: eventvkey."Left" ("VKey") -> [w364 _]
          frame "Left", "Right" {
            n242 = Equal?(x=w364, y=w366) -> (x = y?=w365:bool)
            n243 = Select(t=0, s=w365, f=1) -> (s? t:f=w367:i32)
            n244 = property on="CheckList" class="LstBox (strict)"() -> ("Item Symbols"=w370:i32[])  [unwired: 2 in, 2 out]
            n245 = Replace Array Subset(array=w370, new element=w367, index="CheckList") -> (w369:i32[])
            n246 = property on="CheckList" class="LstBox (strict)"("Item Symbols"=w369) -> ()  [unwired: 2 in, 2 out]
          }
          frame Default {
          }
        }
      }
      event "Motor.Enable": Value Change {
        # "When the test mode otor enable helper is set, update that\ntree row item's value"
        n247 = event-data() -> ("NewVal"=w375:bool)  [unwired: 1 in]
        n248 = Unbundle("Motor") -> ("Value"=w374:dbl)  [unwired: 1 out]
        n249 = Select(t=w374, s=w375, f=0.0) -> (s? t:f=w372:dbl)
        n250 = call <vilib>:"NT Write Number.vi"("value"=w372, "name"=w371) -> ()  [unwired: 9 in, 1 out]
      }
      event "Test Slider": Value Change {
        # "When the test mode slider helper is set, update that\ntree row item's value"
        n251 = event-data() -> ("NewVal"=w377:dbl)  [unwired: 1 in]
        n252 = call <vilib>:"NT Write Number.vi"("value"=w377, "name"=w378) -> ()  [unwired: 9 in, 1 out]
      }
      event "On/Off": Value Change {
        # "When the test mode on/off helper value is set, update that\ntree row item's value"
        n253 = event-data() -> ("NewVal"=w381:bool)  [unwired: 1 in]
        n254 = Boolean To (0,1)(Boolean=w381) -> (0, 1=w380:i16)
        n255 = call <vilib>:"NT Write Number.vi"("value"=w380, "name"=w379) -> ()  [unwired: 9 in, 1 out]
      }
      event "Rev/Fwd": Value Change {
        # "When the test mode helper value for relays is set, update that\ntree row item's value"
        n256 = event-data() -> ("NewVal.Forward"=w388:bool, "NewVal.Reverse"=w387:bool)  [unwired: 1 in]
        n257 = Boolean To (0,1)(Boolean=w388) -> (0, 1=w384:i16)
        n258 = Boolean To (0,1)(Boolean=w387) -> (0, 1=w386:i16)
        n259 = Negate(x=w386) -> (-x=w385:i16)
        n260 = Add(x=w384, y=w385) -> (x+y=w383:i16)
        n261 = call <vilib>:"NT Write Number.vi"("value"=w383, "name"=w382) -> ()  [unwired: 9 in, 1 out]
      }
      event "Test Ring": Value Change {
        # "When a test mode helper value is selected from the ring,\nset the tree item's variable to the string value"
        n262 = event-data() -> ("NewVal"=w391:u16)  [unwired: 1 in]
        n263 = property on="Test Ring" class="Ring (strict)"() -> ("Strings []"=w392:string[])  [unwired: 2 in, 2 out]
        n264 = Index Array(array=w392, index=w391) -> (element=w390:string)
        n265 = call <vilib>:"NT Write String.vi"("value"=w390, "name"=w389) -> ()  [unwired: 9 in, 1 out]
      }
      event "Rec Mode": Value Change {
        # "Update globals for recording mode and path to read log from.\nClear when logging and let NetworkTables set path for vision to\nuse."
        n266 = event-data() -> ("NewVal"=w401:enum32{"Stop", "Record", "Playback"})  [unwired: 1 in]
        n267 = global write "WPI_DashboardLogging Global.vi" "Logging Filename"(path "") -> ()
        n268 = global write "WPI_DashboardLogging Global.vi" "Recording"(w401) -> ()
        n269 = case shown="\"Playback\"" w401 {
          tunnel: w400 -> [_ w403 w411]
          tunnel: [_ _ w410] -> w398
          tunnel: [_ _ w409] -> _
          tunnel: w396 -> [_ _ w407]
          tunnel: cluster{i32, i32} {-250, 170} -> [_ _ w406]
          tunnel: [_ _ T27 {"Image Size"=TRUE, "Image Type"=TRUE, "Pixel Value"=TRUE, "ROI Information"=TRUE, "Zoom Factor"=FALSE} ("Image Information Shown:All Elements")] -> w393
          tunnel: [_ _ TRUE ("Zoom Factor")] -> w394
          frame Default {
          }
          frame "Stop", "Record" {
            # "Place Window too"
            n270 = invoke class="VI" method="FP.Close"(reference=w403) -> (reference out=w402:refnum<vi>)  [unwired: 2 in, 2 out]
            n271 = invoke class="VI" method="Abort VI"(reference=w402) -> ()  [unwired: 2 in, 3 out]
          }
          frame "Playback" {
            n272 = call "Open Playback Panel.vi"("Offset"=w406, "DB VI Ref"=w407, "Playback in"=w411) -> ("Playback out"=w408:refnum<vi>)  [unwired: 8 in]
            n273 = register-events(w408) -> (reference out=w410:refnum<event-registration>, error out=w409:errorcluster)  [unwired: 2 in]
          }
        }
        n274 = property on="Camera Image Right" class="ImageControl"("Image Information Shown"=w393, "Image Information Visible"=w394) -> ()  [unwired: 2 in, 2 out]
        n275 = property on="Camera Image" class="ImageControl"("Image Information Shown"=w393, "Image Information Visible"=w394) -> ()  [unwired: 2 in, 2 out]
        n276 = call <vilib>:"WPI_DashboardNT Log FieldName Cache.vi"("Operation"=enum16{"Lookup/Add", "Index", "Clear"}."Clear") -> ()  [unwired: 8 in, 3 out]
      }
      event Panel Close {
        w412 = enum32{"Stop", "Record", "Playback"}."Stop" ("Rec Mode")
        # "Playback window has been closed, abort"
        n277 = event-data() -> ()  [unwired: 1 in, 4 out]
        n278 = local write "Rec Mode"(w412) -> ()
        n279 = global write "WPI_DashboardLogging Global.vi" "Recording"(w412) -> ()
      }
      event Panel Close {
        # "Abort playback window and ourself"
        n280 = event-data() -> ()  [unwired: 1 in, 4 out]
        n281 = invoke class="VI" method="FP.Close"(reference=w415) -> (reference out=w414:refnum<vi>)  [unwired: 2 in, 2 out]
        n282 = invoke class="VI" method="Abort VI"(reference=w414) -> (error out=w413:errorcluster)  [unwired: 2 in, 2 out]
        n283 = invoke class="VI" method="Abort VI"(error in=w413) -> ()  [unwired: 2 in, 3 out]
      }
      event "Tree": Double Click {
        n284 = event-data() -> ("PlatMods"=w421:T29, "Tag"=w418:string)  [unwired: 1 in]
        n285 = Unbundle(w421) -> ("Shift"=w420:bool)  [unwired: 4 out]
        n286 = String Subset(string=w418, length (rest)=1 ("length (rest)")) -> (substring=w417:string)  [unwired: 1 in]
        n287 = Not(x=w420) -> (.not. x?=w419:bool)
        n288 = case shown="\"/\"" w417 {
          tunnel: w418 -> [_ w423]
          tunnel: w419 -> [_ w422]
          frame Default {
          }
          frame "/" {
            n289 = call <vilib>:"NT Update Persistence.vi"("Persistence"=w422, "Name"=w423) -> ()  [unwired: 9 in, 1 out]
          }
        }
      }
    }
  }
  n290 = while {
    tunnel: w59 -> [w425]
    i -> [w428]
    stop <- FALSE stop-if-true
    n291 = Wait (ms)(milliseconds to wait=u32 100) -> ()  [unwired: 1 out]
    n292 = case shown="\"Playback\"" "Rec Mode" {
      tunnel: w428 -> [_ _ w443]
      tunnel: [u32 2829099 ("Base Color") u32 11141120 ("Target Color") w432] -> w424
      frame "Stop", Default {
        # "Reset the color, extra updates don't cost much"
      }
      frame "Record" {
      }
      frame "Playback" {
        # "Playback"
        n293 = Quotient & Remainder(x=w443, y=u32 50 ("milliseconds to wait")) -> (x-y*floor(x/y)=w439:u32)  [unwired: 1 out]
        n294 = Divide(x=w439, y=u32 50 ("milliseconds to wait")) -> (x/y=w436:dbl)
        n295 = Multiply(x=6.283185307179586, y=w436) -> (x*y=w441:dbl)
        n296 = Sine(x=w441) -> (sin(x)=w440:dbl)
        n297 = Absolute Value(x=w440) -> (abs(x)=w433:dbl)
        n298 = call "Interpolate RGB Color.vi"("Proportion"=w433, "Target Color"=u32 30976, "Base Color"=u32 2829099) -> ("Result Color"=w432:u32)  [unwired: 8 in]
      }
    }
    n299 = property class="Pane"(reference=w425, "PaneColor"=w424) -> ()  [unwired: 1 in, 2 out]
  }
  n300 = local write "Dashboard Tab"(T9."Drive" ("Dashboard Tab")) -> ()
  n301 = call <vilib>:"Read PNG File.vi"("path to PNG file"="path to PNG file") -> ("image data"=w2:T30)  [unwired: 8 in, 2 out]
  n302 = call <vilib>:"Draw Flattened Pixmap.vi"("image data"=w2) -> ("new picture"=w3:picture)  [unwired: 8 in]
  n303 = property on="On/Off" class="Bool (strict)"("Visible"=w31) -> ()  [unwired: 2 in, 2 out]
  n304 = property on="Motor" class="Clust (strict)"("Visible"=w31) -> ()  [unwired: 2 in, 2 out]
  n305 = property on="Progress" class="Clust (strict)"("Visible"=w31) -> ()  [unwired: 2 in, 2 out]
  n306 = property on="Test Ring" class="Ring (strict)"("Visible"=w31) -> ()  [unwired: 2 in, 2 out]
  n307 = property on="Rev/Fwd" class="Clust (strict)"("Visible"=w31) -> ()  [unwired: 2 in, 2 out]
  n308 = property on="XY Graph" class="XYGraph (strict)"("Plot.Point Style"=u8 2, "Plot.Plot Interpolation"=u8 0, "PlotImages.Back"=w3) -> ()  [unwired: 2 in, 2 out]
  n309 = while {
    tunnel: u16 1741 ("timeout ms (25000)") -> [w445]
    stop <- FALSE stop-if-true
    n310 = TCP Create Listener(10:w445) -> (0:w444:errorcluster, 3:w446:refnum<k5>)  [unwired: 4 in, 1 out]
    n311 = case shown="No Error" w444 {
      selector: w444 -> [w448 _]
      tunnel: w446 -> [w449 _]
      frame No Error {
        n312 = while {
          tunnel: w449 -> [w452]
          tunnel: w448 -> [w451]
          stop <- FALSE stop-if-true
          n313 = TCP Wait On Listener(8:w451, 11:w452) -> (0:w453:errorcluster, 4:w454:refnum<k5>)  [unwired: 2 in, 3 out]
          n314 = local write "TCP"(w454) -> ()
          n315 = case shown="Error" w453 {
            frame No Error {
            }
            frame Error {
              n316 = Wait (ms)(milliseconds to wait=u32 1000) -> ()  [unwired: 1 out]
            }
          }
        }
      }
      frame Error {
        n317 = Wait (ms)(milliseconds to wait=u32 1000) -> ()  [unwired: 1 out]
      }
    }
  }
  n318 = global write "WPI_DashboardLogging Global.vi" "Recording"(w54) -> ()
  n319 = local write "Rec Mode"(w54) -> ()
  n320 = call <vilib>:"NT Write String.vi"("value"="Select Auto", "name"="Auto Selector" ("Name")) -> ()  [unwired: 9 in, 1 out]
